vi "CThread Decode CThread Reference.vi"(2 "Owner Path":path, 3 "CThread Reference":string) -> (0 "Clone Number":i16, 1 "path":path)   [LabVIEW 2012, in "CThread.lvlib"]
uses:
  CThread.lvlib
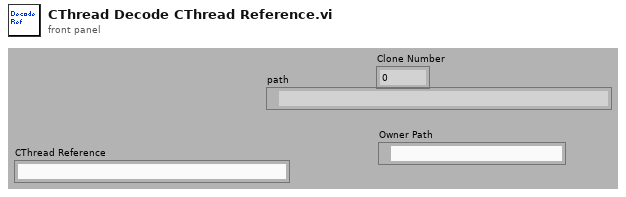
[diagram p1: front panel]
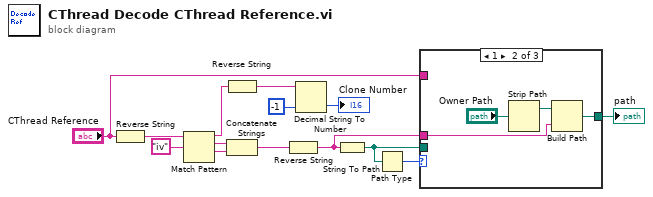
[diagram p0: block diagram]
diagram:
  n1 = Reverse String(1:"CThread Reference") -> (0:w13:string)
  n2 = Match Pattern(string=w13, regular expression="iv") -> (before substring=w1:string, match substring=w10:string, after substring=w11:string)  [unwired: 1 in, 1 out]
  n3 = Reverse String(1:w1) -> (0:w2:string)
  n4 = Concatenate Strings(w10, w11) -> (w9:string)
  n5 = Reverse String(1:w9) -> (0:w8:string)
  n6 = Decimal String To Number(string=w2, default (0L)=i16 -1 ("default (0 I32)")) -> (number=→"Clone Number":i16)  [unwired: 1 in, 1 out]
  n7 = String To Path(string=w8) -> (path=w6:path)
  n8 = Path Type(1:w6) -> (0:w12:i16)
  n9 = case shown="1" w12 {
    tunnel: w8 -> [_ w17 _]
    tunnel: [w15 w16 _] -> w7
    tunnel: w6 -> [w15 _ _]
    tunnel: "CThread Reference" -> [_ _ _]
    frame 0 {
    }
    frame 1 {
      n10 = Strip Path(path="Owner Path") -> (stripped path=w18:path)  [unwired: 1 out]
      n11 = Build Path(base path=w18, name or relative path=w17) -> (appended path=w16:path)
    }
    frame Default {
    }
  }
  "path" <- w7
